vi "WriteTxt2d.vi"() -> ()   [LabVIEW 2014]
panel:
  in  "Path":path
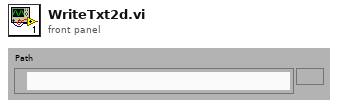
[diagram p1: front panel]
types:
  T1 = enum16{"open", "replace", "create", "open or create", "replace or create", "replace or create with confirmation"}
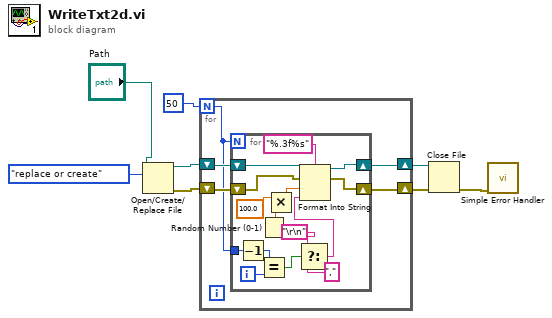
[diagram p0: block diagram]
diagram:
  n1 = Open/Create/Replace File(file path (use dialog)="Path", operation (0:open)=T1."replace or create") -> (refnum out=w7:refnum<file>, error out=w6:errorcluster)  [unwired: 4 in, 1 out]
  n2 = for {
    N: 50 -> [w11]
    shift-right: [w10] -> w4
    shift-left: w7 -> [w13]
    shift-right: [w9] -> w5
    shift-left: w6 -> [w12]
    n3 = for {
      N: w11 -> [_]
      shift-right: [w26] -> w9
      shift-left: w12 -> [w25]
      shift-right: [w27] -> w10
      shift-left: w13 -> [w28]
      tunnel: w11 -> [w20]
      i -> [w19]
      n4 = Decrement(x=w20) -> (x-1=w18:i32)
      n5 = Random Number (0-1)() -> (number: 0 to 1=w24:dbl)
      n6 = Equal?(x=w18, y=w19) -> (x = y?=w17:bool)
      n7 = Multiply(x=100.0, y=w24) -> (x*y=w22:dbl)
      n8 = Select(t="\r\n", s=w17, f=",") -> (s? t:f=w15:string)
      n9 = Format Into String(format string="%.3f%s", initial string=w28, error in=w25, w22, w15) -> (resulting string=w27:refnum<file>, error out=w26:errorcluster)
    }
  }
  n10 = Close File(refnum=w4, error in=w5) -> (error out=w3:errorcluster)  [unwired: 1 out]
  n11 = call <vilib>:"Simple Error Handler.vi"("error in (no error)"=w3) -> ()  [unwired: 4 in, 5 out]
